vi "Tanslate GPS Data.vi"(8 "East or West":string, 9 "North or South":string, 10 "Longitude Reading":string, 11 "Latitude Reading":string) -> (3 "Direction":dbl, 5 "Longitude":dbl, 7 "Latitude":dbl)   [LabVIEW 2011]
panel:
  out "number 4":dbl
  out "number 3":dbl
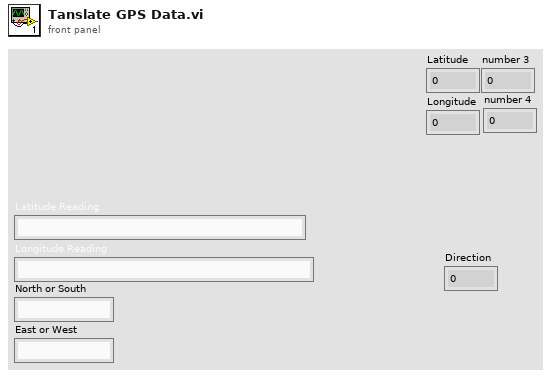
[diagram p1: front panel]
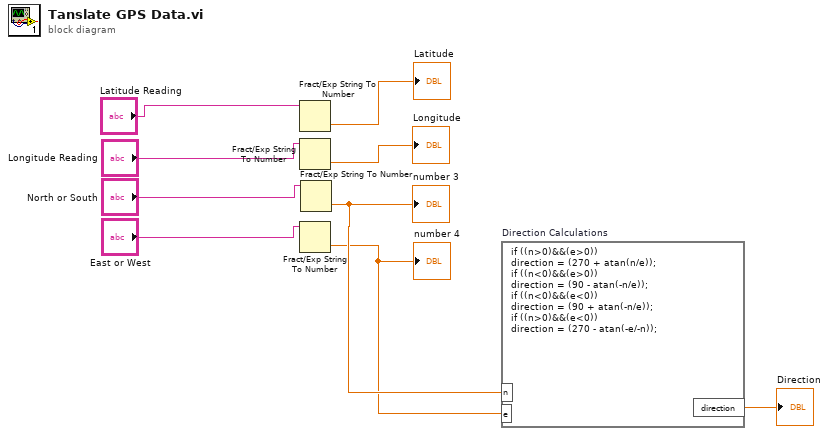
[diagram p0: block diagram]
diagram:
  n1 = Fract/Exp String To Number(string="Latitude Reading") -> (number=→"Latitude":dbl)  [unwired: 3 in, 1 out]
  n2 = Fract/Exp String To Number(string="Longitude Reading") -> (number=→"Longitude":dbl)  [unwired: 3 in, 1 out]
  n3 = Fract/Exp String To Number(string="East or West") -> (number=w2:dbl)  [unwired: 3 in, 1 out]
  "number 4" <- w2
  n4 = Fract/Exp String To Number(string="North or South") -> (number=w3:dbl)  [unwired: 3 in, 1 out]
  "number 3" <- w3
  n5 = formula code="if ((n>0)&&(e>0))\ndirection = (270 + atan(n/e));\nif ((n<0)&&(e>0))\ndirection = (90 - atan(-n/e));\nif ((n<0)&&(e<0))\ndirection = (90 + atan(-n/e));\nif ((n>0)&&(e<0))\ndirection = (270 - atan(-e/-n));" "Direction Calculations"("n"=w3, "e"=w2) -> ("direction"=→"Direction":dbl)
